vi "Send Email Attachment LV 2012 NI Verified.vi"(0 "Email Account ID":string, 4 "Port":i32=25, 5 "Email Account Password":string, 7 "SMTP Outgoing Mail Server":string="smtp.gmail.com", 9 "From: (email@site.com)":string, 11 "To: (email@site.com)":string, 12 "Subject:":string, 13 "Body:":string) -> (15 "MailSuccess":bool)   [LabVIEW 2017]
panel:
  # "Overview: This example shows how to send email attachments from LabVIEW using any SMTP email service, such as Gmail.\nRequirements: LabVIEW 2012 (or compatible)\nInstructions: \n1. Configure all the controls on the front panel. If you use a Gmail account, set SMTP Outgping Mail Server to smtp.gmail.com\n2. Run the VI"
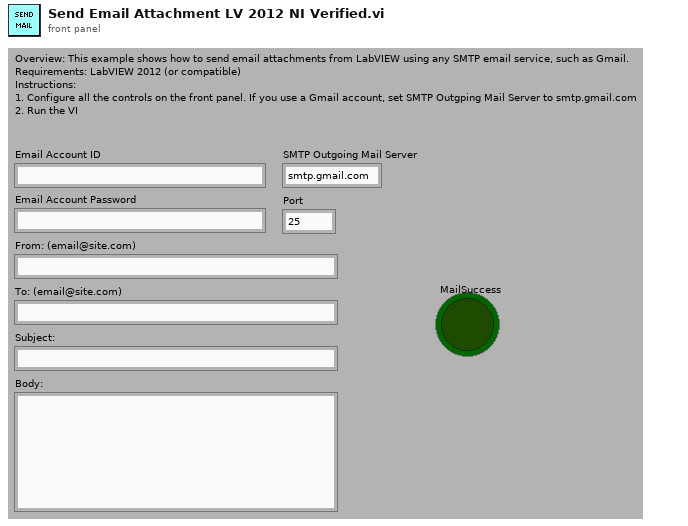
[diagram p1: front panel]
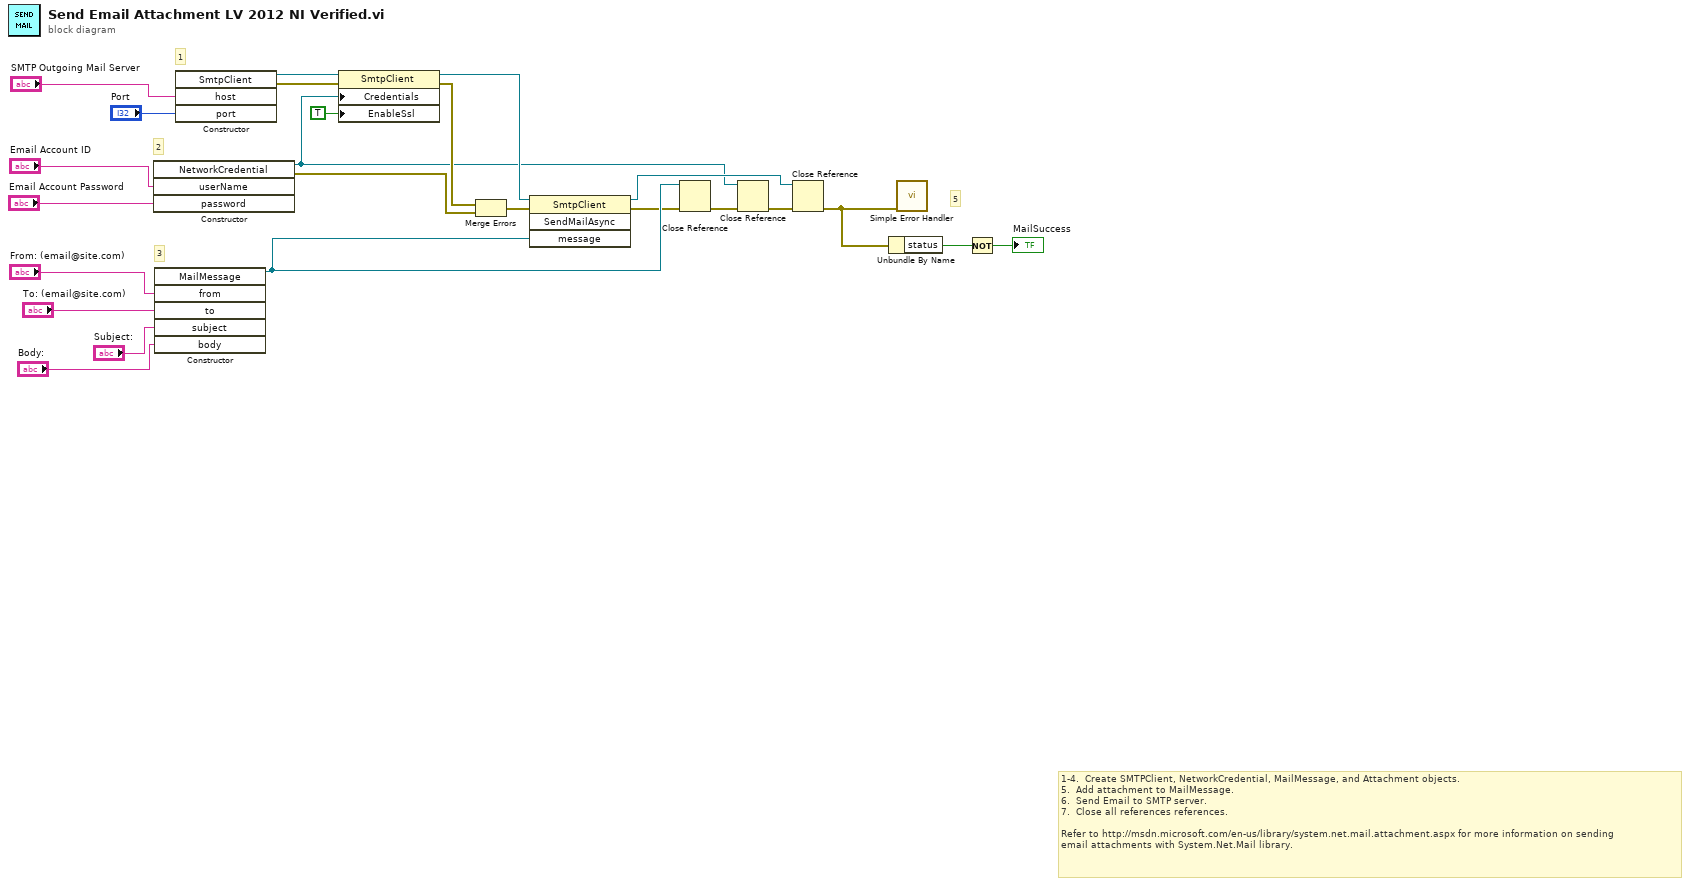
[diagram p0: block diagram]
diagram:
  # "1-4.  Create SMTPClient, NetworkCredential, MailMessage, and Attachment objects.\n5.  Add attachment to MailMessage.\n6.  Send Email to SMTP server.\n7.  Close all references references.\n\nRefer to http://msdn.microsoft.com/en-us/library/system.net.mail.attachment.aspx for more information on sending\nemail attachments with System.Net.Mail library."
  # "5"
  # "3"
  # "2"
  # "1"
  n1 = constructor class="NetworkCredential"("userName"="Email Account ID", "password"="Email Account Password") -> (reference out=w7:refnum<k24>, error out=w9:errorcluster)  [unwired: 3 in, 3 out]
  n2 = constructor class="MailMessage"("from"="From: (email@site.com)", "to"="To: (email@site.com)", "subject"="Subject:", "body"="Body:") -> (reference out=w3:refnum<k24>)  [unwired: 3 in, 6 out]
  n3 = constructor class="SmtpClient"("host"="SMTP Outgoing Mail Server", "port"="Port") -> (reference out=w24:refnum<k24>, error out=w13:errorcluster)  [unwired: 3 in, 3 out]
  n4 = property class="SmtpClient"(reference=w24, error in=w13, "Credentials"=w7, "EnableSsl"=TRUE ("Enable SSL")) -> (reference out=w23:refnum<k24>, error out=w12:errorcluster)
  n5 = Merge Errors(w12, w9) -> (w11:errorcluster)
  n6 = invoke class="SmtpClient" method="SendMailAsync"(reference=w23, error in=w11, "message"=w3) -> (reference out=w10:refnum<k24>, error out=w1:errorcluster)  [unwired: 1 in, 2 out]
  n7 = Close Reference(reference=w3, error in (no error)=w1) -> (error out=w8:errorcluster)
  n8 = Close Reference(reference=w7, error in (no error)=w8) -> (error out=w6:errorcluster)
  n9 = Close Reference(reference=w10, error in (no error)=w6) -> (error out=w2:errorcluster)
  n10 = Unbundle By Name(w2) -> ("status"=w5:bool)
  n11 = call <vilib>:"Simple Error Handler.vi"("error in (no error)"=w2) -> ()  [unwired: 4 in, 5 out]
  n12 = Not(x=w5) -> (.not. x?=→"MailSuccess":bool)
